vi "MMControl.vi"(5 "MM System":u16(ring) items=["MM3000", "MM2000"]) -> ()   [LabVIEW 2022 SP3]
uses:
  -MotionRoutines/MotionGlobals.vi
  MM2KRRI.llx/Power ON/OFF.vi
panel:
  in  "Z Position (mm)":dbl format="%.3f"
  in  "FineMi3":bool
  in  "FinePl3":bool
  in  "Rst3":bool
  in  "Ax3Plus":bool
  in  "Ax3Minus":bool
  in  "Y Position (mm)":dbl format="%.3f"
  in  "FineMi2":bool
  in  "FinePl2":bool
  in  "Rst2":bool
  in  "Ax2Plus":bool
  in  "Ax2Minus":bool
  in  "X Position (mm)":dbl format="%.3f"
  in  "stop":bool
  in  "FineMi1":bool
  in  "FinePl1":bool
  in  "Rst1":bool
  in  "Ax1Plus":bool
  in  "Ax1Minus":bool
  # "Units are in mm. \"Rst\" zeros the position. Blue circles move 1 cm for linear, 360 degrees for rotational."
  # "X Axis"
  # "Y Axis"
  # "Z Axis"
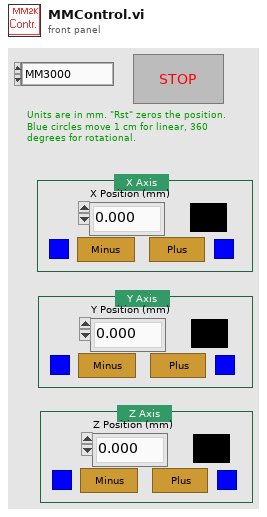
[diagram p1: front panel]
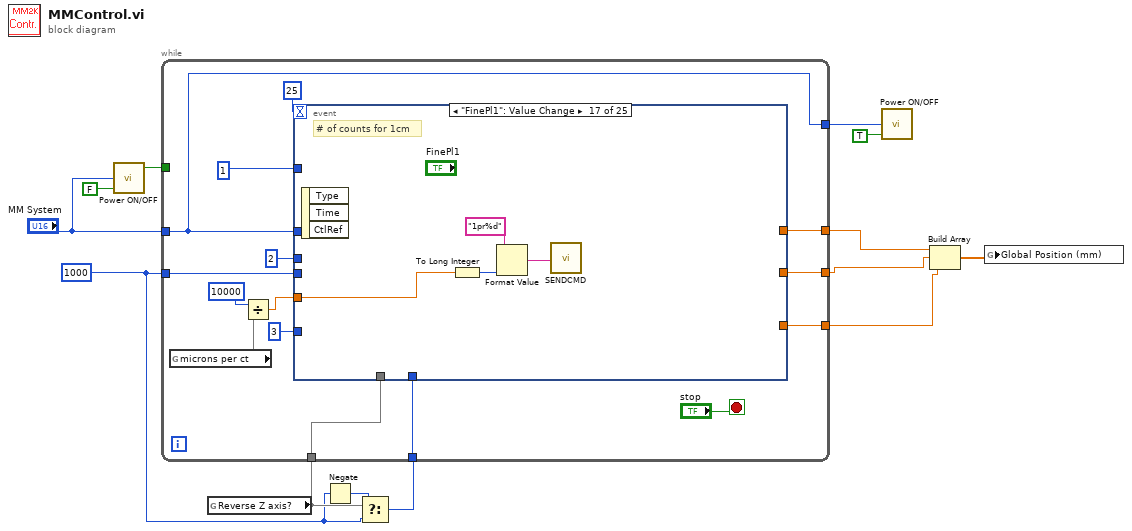
[diagram p0: block diagram]
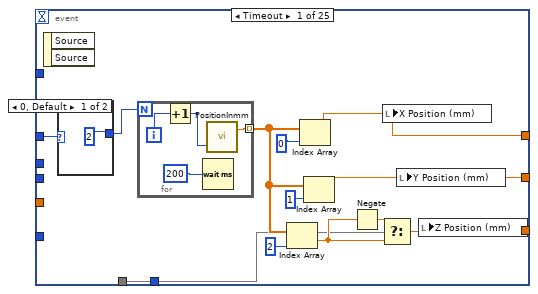
[diagram p2: hidden frame]
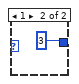
[diagram p3: hidden frame]
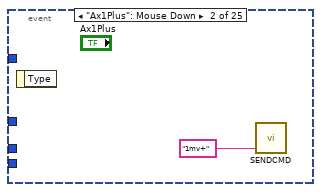
[diagram p4: hidden frame]
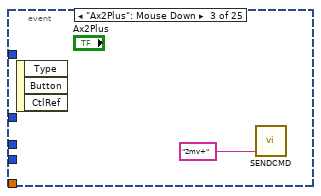
[diagram p5: hidden frame]
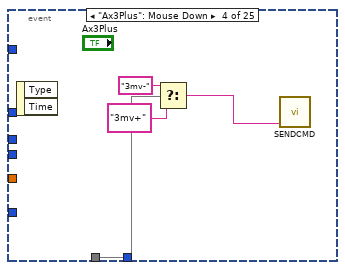
[diagram p6: hidden frame]
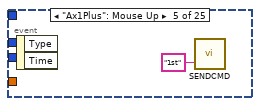
[diagram p7: hidden frame]
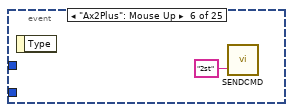
[diagram p8: hidden frame]
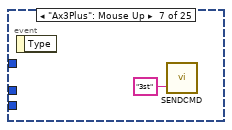
[diagram p9: hidden frame]
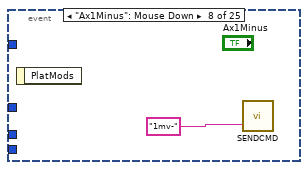
[diagram p10: hidden frame]
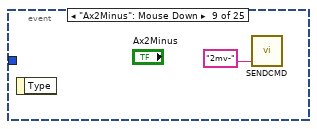
[diagram p11: hidden frame]
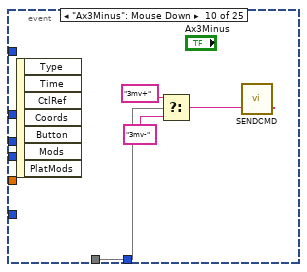
[diagram p12: hidden frame]
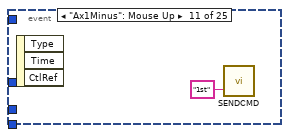
[diagram p13: hidden frame]
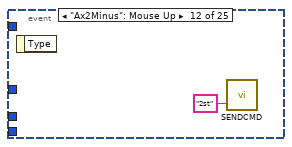
[diagram p14: hidden frame]
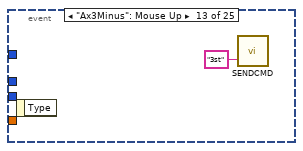
[diagram p15: hidden frame]
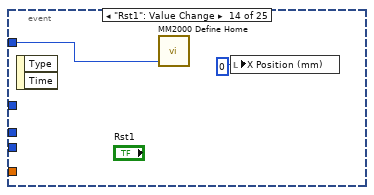
[diagram p16: hidden frame]
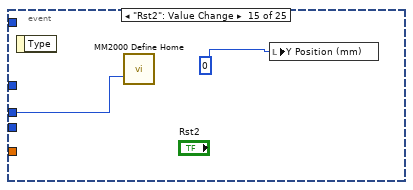
[diagram p17: hidden frame]
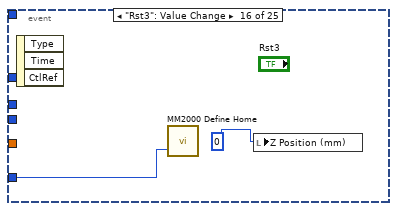
[diagram p18: hidden frame]
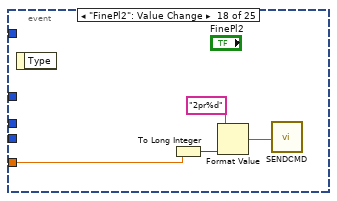
[diagram p19: hidden frame]
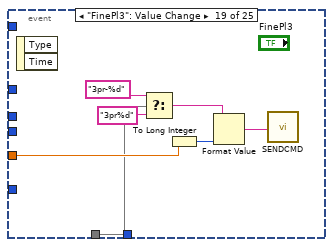
[diagram p20: hidden frame]
diagram:
  w10 = 1000 ("y")
  n1 = call "Power ON/OFF.vi"("OFF (T)/ON (F)"=FALSE, "MM System"="MM System") -> ("Error"=w9:bool)  [unwired: 3 in]
  n2 = global read "MotionGlobals.vi" "Reverse Z axis?"() -> (w11)
  n3 = Negate(x=w10) -> (-x=w13:i32)
  n4 = Select(t=w13, s=w11, f=w10) -> (s? t:f=w12:i32)
  n5 = while {
    tunnel: w12 -> [w27]
    tunnel: w11 -> [w22]
    tunnel: "MM System" -> [w14]
    tunnel: [w26] -> w4
    tunnel: [w25] -> w3
    tunnel: [w24] -> w2
    tunnel: w10 -> [w18]
    tunnel: w9 -> [_]
    tunnel: [w14] -> w6
    stop <- "stop" stop-if-true
    n6 = global read "MotionGlobals.vi" "microns per ct"() -> (w15)
    n7 = Divide(x=10000, y=w15) -> (x/y=w16:dbl)
    n8 = event shown="[16] \"FinePl1\": Value Change" {
      selector: _ -> [_ _ _ _ _ _ _ _ _ _ _ _ _ _ _ _ _ _ _ _ _ _ _ _ _]
      dyn-events: _ -> [_ _ _ _ _ _ _ _ _ _ _ _ _ _ _ _ _ _ _ _ _ _ _ _ _]
      timeout: 25 -> [_ _ _ _ _ _ _ _ _ _ _ _ _ _ _ _ _ _ _ _ _ _ _ _ _]
      tunnel: w27 -> [_ _ _ _ _ _ _ _ _ _ _ _ _ _ _ _ _ _ _ _ _ _ _ _ w112]
      tunnel: 1 -> [_ _ _ _ _ _ _ _ _ _ _ _ _ w65 _ _ _ _ _ _ _ _ w102 _ _]
      tunnel: w22 -> [w29 _ _ w51 _ _ _ _ _ w59 _ _ _ _ _ _ _ _ w79 _ _ w95 _ _ _]
      tunnel: 2 -> [_ _ _ _ _ _ _ _ _ _ _ _ _ _ w67 _ _ _ _ _ _ _ _ w107 _]
      tunnel: 3 -> [_ _ _ _ _ _ _ _ _ _ _ _ _ _ _ w69 _ _ _ _ _ _ _ _ w109]
      tunnel: w16 -> [_ _ _ _ _ _ _ _ _ _ _ _ _ _ _ _ w71 w75 w83 w86 w90 w94 _ _ _]
      tunnel: w14 -> [w33 _ _ _ _ _ _ _ _ _ _ _ _ _ _ _ _ _ _ _ _ _ _ _ _]
      tunnel: [w32 _ _ _ _ _ _ _ _ _ _ _ _ _ _ _ _ _ _ _ _ _ _ _ _] -> w26
      tunnel: [w31 _ _ _ _ _ _ _ _ _ _ _ _ _ _ _ _ _ _ _ _ _ _ _ _] -> w25
      tunnel: [w30 _ _ _ _ _ _ _ _ _ _ _ _ _ _ _ _ _ _ _ _ _ _ _ _] -> w24
      tunnel: w18 -> [_ _ _ _ _ _ _ _ _ _ _ _ _ _ _ _ _ _ _ _ _ _ w101 w106 _]
      event Timeout {
        n9 = event-data() -> ()  [unwired: 3 out]
        n10 = case shown="0, Default" w33 {
          tunnel: [2 3] -> w34
          frame 0, Default {
          }
          frame 1 {
          }
        }
        n11 = for {
          N: w34 -> [_]
          tunnel: [w44] -> w39 mode=indexing
          i -> [w46]
          n12 = Increment(x=w46) -> (x+1=w45:i32)
          n13 = Wait (ms)(milliseconds to wait=200) -> ()  [unwired: 1 out]
          n14 = call "PositionInmm.vi"("Axis"=w45) -> ("postion in mm"=w44:dbl)  [unwired: 1 in, 1 out]
        }
        n15 = Index Array(array=w39, index=2 ("Axis")) -> (element=w35:dbl)
        n16 = Index Array(array=w39, index=0 ("Index")) -> (element=w32:dbl)
        n17 = Index Array(array=w39, index=1 ("Axis")) -> (element=w31:dbl)
        n18 = Negate(x=w35) -> (-x=w36:dbl)
        n19 = Select(t=w36, s=w29, f=w35) -> (s? t:f=w30:dbl)
        n20 = local write "X Position (mm)"(w32) -> ()
        n21 = local write "Y Position (mm)"(w31) -> ()
        n22 = local write "Z Position (mm)"(w30) -> ()
      }
      event "Ax1Plus": Mouse Down {
        n23 = event-data() -> ()  [unwired: 2 out]
        n24 = call "SENDCMD.VI"("MM2000 Command (ASCII String)"="1mv+") -> ()  [unwired: 2 in, 1 out]
      }
      event "Ax2Plus": Mouse Down {
        n25 = event-data() -> ()  [unwired: 4 out]
        n26 = call "SENDCMD.VI"("MM2000 Command (ASCII String)"="2mv+") -> ()  [unwired: 2 in, 1 out]
      }
      event "Ax3Plus": Mouse Down {
        n27 = event-data() -> ()  [unwired: 3 out]
        n28 = Select(t="3mv-", s=w51, f="3mv+") -> (s? t:f=w49:string)
        n29 = call "SENDCMD.VI"("MM2000 Command (ASCII String)"=w49) -> ()  [unwired: 2 in, 1 out]
      }
      event "Ax1Plus": Mouse Up {
        n30 = event-data() -> ()  [unwired: 3 out]
        n31 = call "SENDCMD.VI"("MM2000 Command (ASCII String)"="1st") -> ()  [unwired: 2 in, 1 out]
      }
      event "Ax2Plus": Mouse Up {
        n32 = event-data() -> ()  [unwired: 2 out]
        n33 = call "SENDCMD.VI"("MM2000 Command (ASCII String)"="2st") -> ()  [unwired: 2 in, 1 out]
      }
      event "Ax3Plus": Mouse Up {
        n34 = event-data() -> ()  [unwired: 2 out]
        n35 = call "SENDCMD.VI"("MM2000 Command (ASCII String)"="3st") -> ()  [unwired: 2 in, 1 out]
      }
      event "Ax1Minus": Mouse Down {
        n36 = event-data() -> ()  [unwired: 2 out]
        n37 = call "SENDCMD.VI"("MM2000 Command (ASCII String)"="1mv-") -> ()  [unwired: 2 in, 1 out]
      }
      event "Ax2Minus": Mouse Down {
        n38 = event-data() -> ()  [unwired: 2 out]
        n39 = call "SENDCMD.VI"("MM2000 Command (ASCII String)"="2mv-") -> ()  [unwired: 2 in, 1 out]
      }
      event "Ax3Minus": Mouse Down {
        n40 = event-data() -> ()  [unwired: 8 out]
        n41 = Select(t="3mv+", s=w59, f="3mv-") -> (s? t:f=w58:string)
        n42 = call "SENDCMD.VI"("MM2000 Command (ASCII String)"=w58) -> ()  [unwired: 2 in, 1 out]
      }
      event "Ax1Minus": Mouse Up {
        n43 = event-data() -> ()  [unwired: 4 out]
        n44 = call "SENDCMD.VI"("MM2000 Command (ASCII String)"="1st") -> ()  [unwired: 2 in, 1 out]
      }
      event "Ax2Minus": Mouse Up {
        n45 = event-data() -> ()  [unwired: 2 out]
        n46 = call "SENDCMD.VI"("MM2000 Command (ASCII String)"="2st") -> ()  [unwired: 2 in, 1 out]
      }
      event "Ax3Minus": Mouse Up {
        n47 = event-data() -> ()  [unwired: 2 out]
        n48 = call "SENDCMD.VI"("MM2000 Command (ASCII String)"="3st") -> ()  [unwired: 2 in, 1 out]
      }
      event "Rst1": Value Change {
        n49 = event-data() -> ()  [unwired: 3 out]
        n50 = call "MM2000 Define Home.vi"("Axis"=w65) -> ()  [unwired: 1 in]
        n51 = local write "X Position (mm)"(0 ("Primary Reset Position (0)")) -> ()
      }
      event "Rst2": Value Change {
        n52 = event-data() -> ()  [unwired: 2 out]
        n53 = call "MM2000 Define Home.vi"("Axis"=w67) -> ()  [unwired: 1 in]
        n54 = local write "Y Position (mm)"(0 ("Primary Reset Position (0)")) -> ()
      }
      event "Rst3": Value Change {
        n55 = event-data() -> ()  [unwired: 4 out]
        n56 = call "MM2000 Define Home.vi"("Axis"=w69) -> ()  [unwired: 1 in]
        n57 = local write "Z Position (mm)"(0 ("Primary Reset Position (0)")) -> ()
      }
      event "FinePl1": Value Change {
        # "# of counts for 1cm"
        n58 = event-data() -> ()  [unwired: 4 out]
        n59 = To Long Integer(number=w71) -> (32bit integer=w72:i32)
        n60 = Format Value(format string="1pr%d", value (0)=w72) -> (output string=w73:string)  [unwired: 1 out]
        n61 = call "SENDCMD.VI"("MM2000 Command (ASCII String)"=w73) -> ()  [unwired: 2 in, 1 out]
      }
      event "FinePl2": Value Change {
        n62 = event-data() -> ()  [unwired: 2 out]
        n63 = To Long Integer(number=w75) -> (32bit integer=w76:i32)
        n64 = Format Value(format string="2pr%d", value (0)=w76) -> (output string=w77:string)  [unwired: 1 out]
        n65 = call "SENDCMD.VI"("MM2000 Command (ASCII String)"=w77) -> ()  [unwired: 2 in, 1 out]
      }
      event "FinePl3": Value Change {
        n66 = event-data() -> ()  [unwired: 3 out]
        n67 = Select(t="3pr-%d", s=w79, f="3pr%d") -> (s? t:f=w80:string)
        n68 = To Long Integer(number=w83) -> (32bit integer=w84:i32)
        n69 = Format Value(format string=w80, value (0)=w84) -> (output string=w85:string)  [unwired: 1 out]
        n70 = call "SENDCMD.VI"("MM2000 Command (ASCII String)"=w85) -> ()  [unwired: 2 in, 1 out]
      }
      event "FineMi1": Value Change {
        # "# of counts for 1cm"
        n71 = event-data() -> ()  [unwired: 4 out]
        n72 = To Long Integer(number=w86) -> (32bit integer=w87:i32)
        n73 = Format Value(format string="1pr-%d", value (0)=w87) -> (output string=w88:string)  [unwired: 1 out]
        n74 = call "SENDCMD.VI"("MM2000 Command (ASCII String)"=w88) -> ()  [unwired: 2 in, 1 out]
      }
      event "FineMi2": Value Change {
        n75 = event-data() -> ()  [unwired: 3 out]
        n76 = To Long Integer(number=w90) -> (32bit integer=w91:i32)
        n77 = Format Value(format string="2pr-%d", value (0)=w91) -> (output string=w92:string)  [unwired: 1 out]
        n78 = call "SENDCMD.VI"("MM2000 Command (ASCII String)"=w92) -> ()  [unwired: 2 in, 1 out]
      }
      event "FineMi3": Value Change {
        n79 = event-data() -> ()  [unwired: 2 out]
        n80 = Select(t="3pr%d", s=w95, f="3pr-%d") -> (s? t:f=w96:string)
        n81 = To Long Integer(number=w94) -> (32bit integer=w99:i32)
        n82 = Format Value(format string=w96, value (0)=w99) -> (output string=w100:string)  [unwired: 1 out]
        n83 = call "SENDCMD.VI"("MM2000 Command (ASCII String)"=w100) -> ()  [unwired: 2 in, 1 out]
      }
      event "X Position (mm)": Value Change {
        n84 = event-data() -> ("NewVal"=w104:dbl)  [unwired: 1 out]
        n85 = Multiply(x=w104, y=w101) -> (x*y=w103:dbl)
        n86 = call "MM2000 Position Absolute.vi"("Position Absolute"=w103, "Axis"=w102) -> ()  [unwired: 1 in]
      }
      event "Y Position (mm)": Value Change {
        n87 = event-data() -> ("NewVal"=w105:dbl)  [unwired: 1 out]
        n88 = Multiply(x=w106, y=w105) -> (x*y=w108:dbl)
        n89 = call "MM2000 Position Absolute.vi"("Position Absolute"=w108, "Axis"=w107) -> ()  [unwired: 1 in]
      }
      event "Z Position (mm)": Value Change {
        n90 = event-data() -> ("NewVal"=w111:dbl)  [unwired: 1 out]
        n91 = Multiply(x=w111, y=w112) -> (x*y=w110:dbl)
        n92 = call "MM2000 Position Absolute.vi"("Position Absolute"=w110, "Axis"=w109) -> ()  [unwired: 1 in]
      }
    }
  }
  n93 = call "Power ON/OFF.vi"("OFF (T)/ON (F)"=TRUE, "MM System"=w6) -> ()  [unwired: 3 in, 1 out]
  n94 = Build Array(w4, w3, w2) -> (w1:dbl[])
  n95 = global write "MotionGlobals.vi" "Global Position (mm)"(w1) -> ()
